vi "Caller.vi"   [LabVIEW 2021]
panel:
  # "Caller"
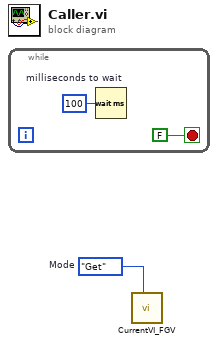
[diagram p0: block diagram]
diagram:
  w1 = enum16{"Get", "Set"}."Get"  # Mode
  n1 = while {
    stop <- FALSE stop-if-true
    w2 = u32 100  # milliseconds to wait
    n2 = Wait (ms)(milliseconds to wait=w2) -> ()  [unwired: 1 out]
  }
  n3 = call "CurrentVI_FGV.vi"("Mode"=w1) -> ()  [unwired: 9 in, 2 out]
